vi "Servo_SetCamera.vi"(2 "error in":errorcluster, 3 "PWM10 Angle in":dbl=nan, 4 "PWM9 Angle in":dbl=nan) -> (0 "error out":errorcluster)   [LabVIEW 2009, in "Servo.lvlib"]
doc: "This function is made to work with the Axis Camera and it's platform. The function assumes that the two servos are at the PWM9 and PWM10. Where PWM9 should be the pitch and PWM10 should be the yaw.\n\nThe values should be in the range of -45 to 45 degrees\n\nThe function takes one or more angels as an input and then sets the camera in that position. If no new angle is presented the servo will stay in its old position for the servo with no input."
uses:
  Servo.lvlib
  PWM/PWM_Name.ctl
  PWM.lvlib
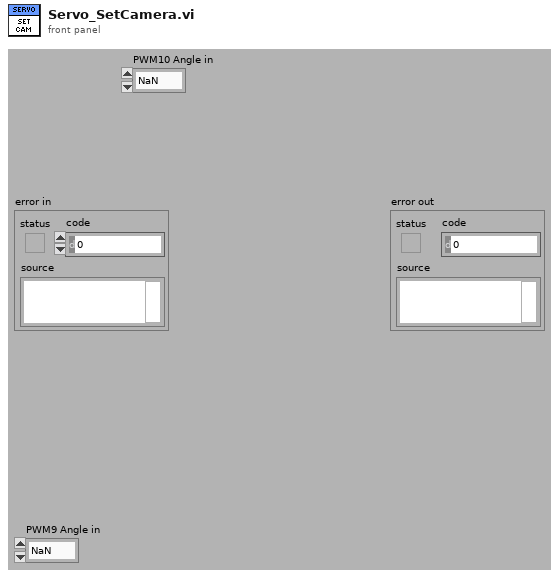
[diagram p1: front panel]
types:
  T1 = typedef "PWM.lvlib/PWM_Name.ctl" = u16
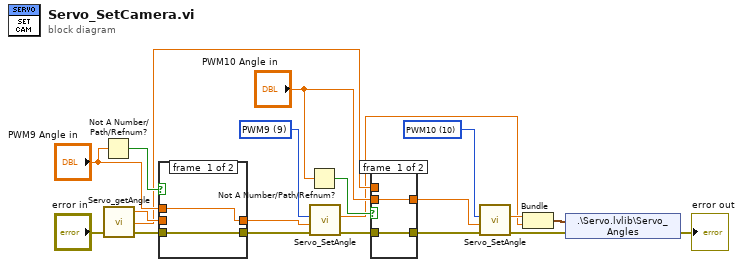
[diagram p0: block diagram]
diagram:
  w9 = T1 10 items=["Invalid"=0, "PWM1"=1, "PWM2"=2, "PWM9"=9, "PWM10"=10] ("PWM")
  w14 = T1 9 items=["Invalid"=0, "PWM1"=1, "PWM2"=2, "PWM9"=9, "PWM10"=10] ("PWM")
  n1 = Not A Number/Path/Refnum?(number/path/refnum="PWM9 Angle in") -> (NaN/Path/Refnum?=w20:bool)
  n2 = call "Servo_getAngle.vi"("error in"="error in") -> ("error out"=w18:errorcluster, "PWM10 Angle"=w7:dbl, "PWM9 Angle"=w17:dbl)  [unwired: 2 in]
  n3 = case shown="False" w20 {
    tunnel: [w22 w24] -> w15
    tunnel: "PWM9 Angle in" -> [w22 _]
    tunnel: w18 -> [w21 w23]
    tunnel: w17 -> [_ w24]
    tunnel: [w21 w23] -> w16
    frame #0 {
    }
    frame #1 {
    }
  }
  n4 = Not A Number/Path/Refnum?(number/path/refnum="PWM10 Angle in") -> (NaN/Path/Refnum?=w13:bool)
  n5 = call "Servo_SetAngle.vi"("error in"=w16, "Angle in"=w15, "PWM"=w14) -> ("error out"=w8:errorcluster, "Angle out"=w5:dbl)  [unwired: 7 in]
  n6 = case shown="False" w13 {
    tunnel: [w26 w28] -> w10
    tunnel: "PWM10 Angle in" -> [w26 _]
    tunnel: w8 -> [w25 w27]
    tunnel: w7 -> [_ w28]
    tunnel: [w25 w27] -> w11
    frame #0 {
    }
    frame #1 {
    }
  }
  n7 = call "Servo_SetAngle.vi"("error in"=w11, "Angle in"=w10, "PWM"=w9) -> ("error out"=w2:errorcluster, "Angle out"=w6:dbl)  [unwired: 7 in]
  n8 = Bundle("Angle out"=w6, "Angle out"=w5) -> (w3:cluster{"Angle out":dbl, "Angle out":dbl})  [unwired: 1 in]
  n9 = shared-variable ".\\Servo.lvlib\\Servo_Angles"(w3, error in=w2) -> (error out=→"error out":errorcluster)
